vi "Process Sink Errors.vi"(8 "error in (no error)":errorcluster[](array[cluster]), 11 "Data Sinks In":refnum<data-value>[](array[refnum])) -> (0 "error out":errorcluster, 3 "Data Sinks Out":refnum<data-value>[](array[refnum]))   [LabVIEW 2017, in "Composed Log.lvlib" / "Application Logger.lvclass"]
uses:
  <vilib>/gpm_packages/@cs/event-logger/Source/Composed Log/Application Logger/Application Logger.lvclass
  <vilib>/gpm_packages/@cs/event-logger/Source/Composed Log/Log Sink/Log Sink.lvclass
  <vilib>/ErrorRing/Error Ring.xnode
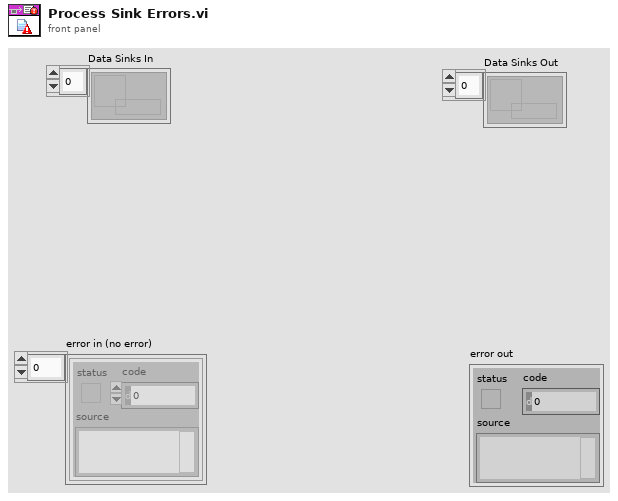
[diagram p1: front panel]
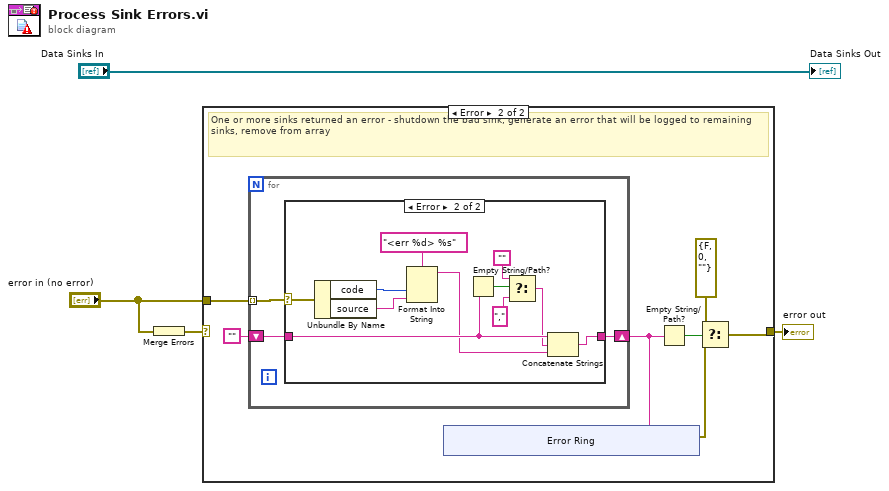
[diagram p0: block diagram]
diagram:
  n1 = Merge Errors("error in (no error)") -> (w4:errorcluster)
  n2 = case shown="Error" w4 {
    selector: w4 -> [w5 _]
    tunnel: "error in (no error)" -> [_ w12]
    tunnel: [w5 w8] -> w2
    frame No Error {
      # "No error - do nothing"
    }
    frame Error {
      # "One or more sinks returned an error - shutdown the bad sink, generate an error that will be logged to remaining sinks, remove from array"
      n3 = for {
        tunnel: w12 -> [w15] mode=indexing
        shift-right: [w13] -> w10
        shift-left: "" -> [w14]
        n4 = case shown="Error" w15 {
          selector: w15 -> [_ w27]
          tunnel: w14 -> [w16 w23]
          tunnel: [w16 w24] -> w13
          frame No Error {
          }
          frame Error {
            n5 = Unbundle By Name(w27) -> ("code"=w26:i32, "source"=w25:string)
            n6 = Format Into String(format string="<err %d> %s", w26, w25) -> (resulting string=w19:string)  [unwired: 2 in, 1 out]
            n7 = Empty String/Path?(string/path=w23) -> (empty?=w21:bool)
            n8 = Select(t="", s=w21, f=",") -> (s? t:f=w20:string)
            n9 = Concatenate Strings(w23, w20, w19) -> (w24:string)
          }
        }
      }
      n10 = xnode "Error Ring"("parameter 0"=w10) -> ("error out"=w6:errorcluster)
      n11 = Empty String/Path?(string/path=w10) -> (empty?=w9:bool)
      n12 = Select(t=errorcluster {"status"=FALSE, "code"=0, "source"=""} ("f"), s=w9, f=w6) -> (s? t:f=w8:errorcluster)
    }
  }
  "error out" <- w2
  "Data Sinks Out" <- "Data Sinks In"
